vi "ResAcc data.vi"() -> ()   [LabVIEW 2013]
panel:
  out "크기":i32[](array[numeric])
  out "웨이브폼 그래프":dbl[][](graph)
  in  "Acc&Res":dbl[][](array[numeric])=array16x2000[32000 elements] caption="가속도, 저항" format="%#.2p"
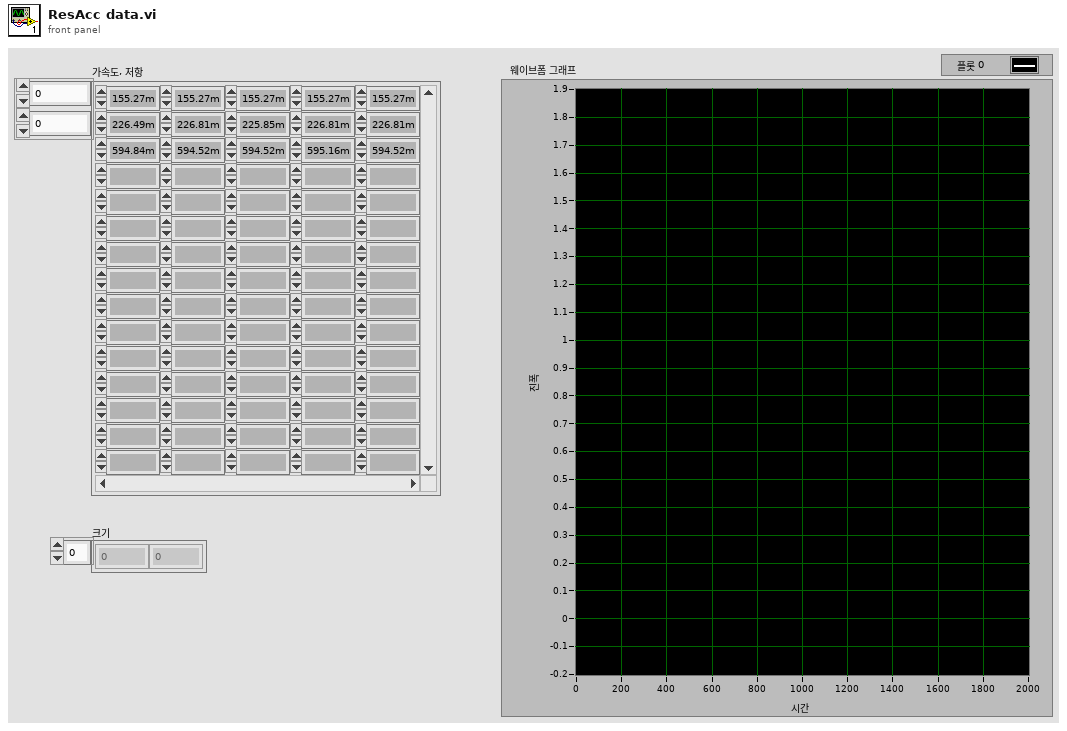
[diagram p1: front panel]
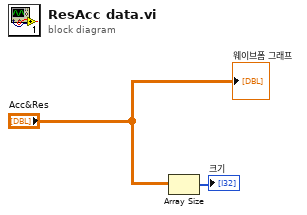
[diagram p0: block diagram]
diagram:
  n1 = Array Size(array="Acc&Res") -> (size(s)=→"크기":i32[])
  "웨이브폼 그래프" <- "Acc&Res"
